vi "TestReadWrites.vi"() -> ()   [LabVIEW 2017]
uses:
  Global 1.vi
panel:
  in  "Indicator 2":dbl
  out "Array":dbl[][](array[numeric])
  out "Indicator":dbl
  out "Time per write":dbl[](array[numeric])
  in  "Iterations":i32=5000
  # "Control/Indicator"
  # "Local Variable"
  # "Property Node"
  # "Global Variable"
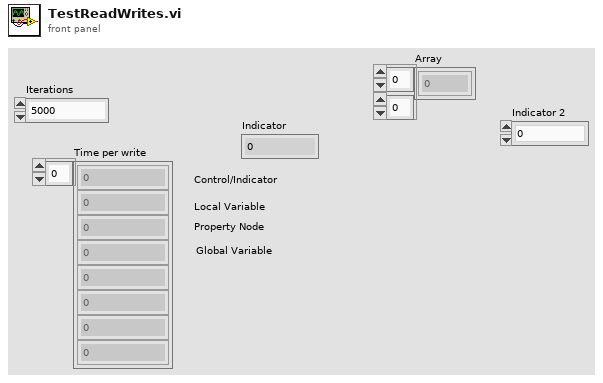
[diagram p1: front panel]
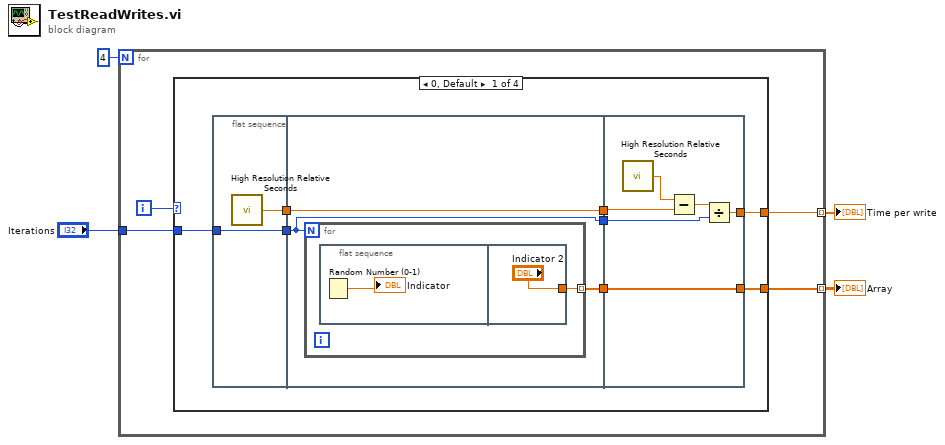
[diagram p0: block diagram]
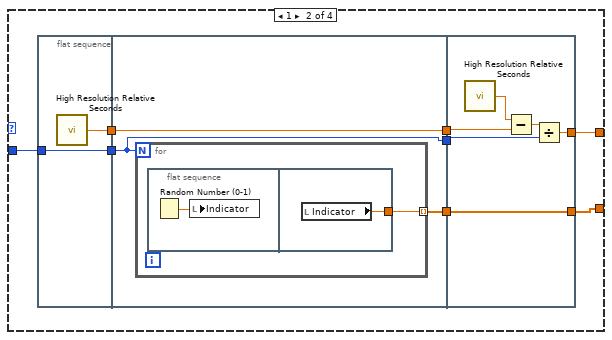
[diagram p2: hidden frame]
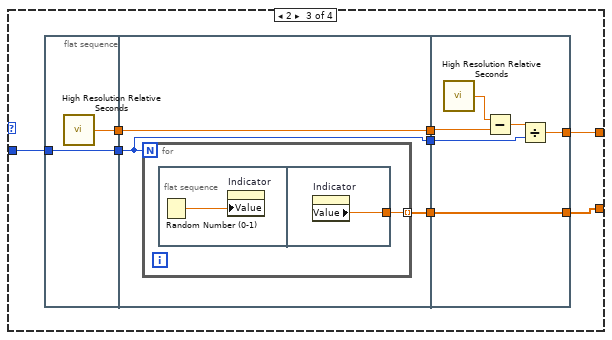
[diagram p3: hidden frame]
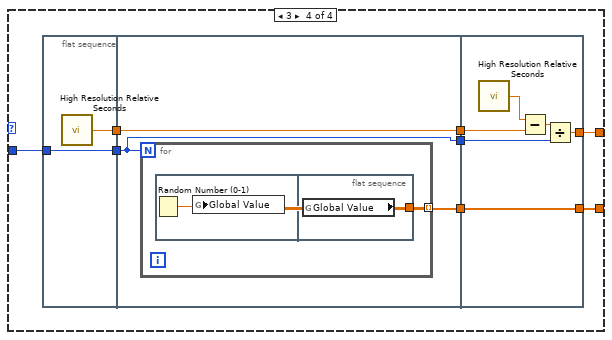
[diagram p4: hidden frame]
diagram:
  n1 = for {
    N: 4 -> [_]
    tunnel: "Iterations" -> [w7]
    tunnel: [w6] -> w3 mode=indexing
    tunnel: [w5] -> w1 mode=indexing
    i -> [w8]
    n2 = case shown="0, Default" w8 {
      tunnel: w7 -> [w14 w36 w58 w80]
      tunnel: [w11 w33 w55 w77] -> w6
      tunnel: [w10 w31 w54 w75] -> w5
      frame 0, Default {
        n3 = flat-sequence {
          tunnel: [w18] -> w15
          tunnel: w14 -> [w17]
          tunnel: [w17] -> w13
          tunnel: [w21] -> w16
          tunnel: w15 -> [w21]
          tunnel: w13 -> [w20]
          tunnel: [w20] -> w12
          tunnel: [w19] -> w9
          tunnel: w16 -> [w29]
          tunnel: w12 -> [w27]
          tunnel: [w26] -> w11
          tunnel: [w25] -> w10
          tunnel: w9 -> [w25]
          frame #0 {
            n4 = call <vilib>:"High Resolution Relative Seconds.vi"() -> ("relative seconds"=w18:dbl)
          }
          frame #1 {
            n5 = for {
              N: w20 -> [_]
              tunnel: [w22] -> w19 mode=indexing
              n6 = flat-sequence {
                tunnel: ["Indicator 2"] -> w22
                frame #0 {
                  n7 = Random Number (0-1)() -> (number: 0 to 1=→"Indicator":dbl)
                }
                frame #1 {
                }
              }
            }
          }
          frame #2 {
            n8 = call <vilib>:"High Resolution Relative Seconds.vi"() -> ("relative seconds"=w30:dbl)
            n9 = Subtract(x=w30, y=w29) -> (x-y=w28:dbl)
            n10 = Divide(x=w28, y=w27) -> (x/y=w26:dbl)
          }
        }
      }
      frame 1 {
        n11 = flat-sequence {
          tunnel: [w40] -> w37
          tunnel: w36 -> [w39]
          tunnel: [w39] -> w35
          tunnel: [w43] -> w38
          tunnel: w37 -> [w43]
          tunnel: w35 -> [w42]
          tunnel: [w42] -> w34
          tunnel: [w41] -> w32
          tunnel: w38 -> [w51]
          tunnel: w34 -> [w49]
          tunnel: [w48] -> w33
          tunnel: [w47] -> w31
          tunnel: w32 -> [w47]
          frame #0 {
            n12 = call <vilib>:"High Resolution Relative Seconds.vi"() -> ("relative seconds"=w40:dbl)
          }
          frame #1 {
            n13 = for {
              N: w42 -> [_]
              tunnel: [w44] -> w41 mode=indexing
              n14 = flat-sequence {
                tunnel: [w46] -> w44
                frame #0 {
                  n15 = Random Number (0-1)() -> (number: 0 to 1=w45:dbl)
                  n16 = local write "Indicator"(w45) -> ()
                }
                frame #1 {
                  n17 = local read "Indicator"() -> (w46:dbl)
                }
              }
            }
          }
          frame #2 {
            n18 = call <vilib>:"High Resolution Relative Seconds.vi"() -> ("relative seconds"=w52:dbl)
            n19 = Subtract(x=w52, y=w51) -> (x-y=w50:dbl)
            n20 = Divide(x=w50, y=w49) -> (x/y=w48:dbl)
          }
        }
      }
      frame 2 {
        n21 = flat-sequence {
          tunnel: [w62] -> w59
          tunnel: w58 -> [w61]
          tunnel: [w61] -> w57
          tunnel: [w65] -> w60
          tunnel: w59 -> [w65]
          tunnel: w57 -> [w64]
          tunnel: [w64] -> w56
          tunnel: [w63] -> w53
          tunnel: w60 -> [w73]
          tunnel: w56 -> [w71]
          tunnel: [w70] -> w55
          tunnel: [w69] -> w54
          tunnel: w53 -> [w69]
          frame #0 {
            n22 = call <vilib>:"High Resolution Relative Seconds.vi"() -> ("relative seconds"=w62:dbl)
          }
          frame #1 {
            n23 = for {
              N: w64 -> [_]
              tunnel: [w66] -> w63 mode=indexing
              n24 = flat-sequence {
                tunnel: [w68] -> w66
                frame #0 {
                  n25 = Random Number (0-1)() -> (number: 0 to 1=w67:dbl)
                  n26 = property on="Indicator" class="DigNum (strict)"("Value"=w67) -> ()  [unwired: 2 in, 2 out]
                }
                frame #1 {
                  n27 = property on="Indicator" class="DigNum (strict)"() -> ("Value"=w68:dbl)  [unwired: 2 in, 2 out]
                }
              }
            }
          }
          frame #2 {
            n28 = call <vilib>:"High Resolution Relative Seconds.vi"() -> ("relative seconds"=w74:dbl)
            n29 = Subtract(x=w74, y=w73) -> (x-y=w72:dbl)
            n30 = Divide(x=w72, y=w71) -> (x/y=w70:dbl)
          }
        }
      }
      frame 3 {
        n31 = flat-sequence {
          tunnel: [w84] -> w81
          tunnel: w80 -> [w83]
          tunnel: [w83] -> w79
          tunnel: [w87] -> w82
          tunnel: w81 -> [w87]
          tunnel: w79 -> [w86]
          tunnel: [w86] -> w78
          tunnel: [w85] -> w76
          tunnel: w82 -> [w95]
          tunnel: w78 -> [w93]
          tunnel: [w92] -> w77
          tunnel: w76 -> [w91]
          tunnel: [w91] -> w75
          frame #0 {
            n32 = call <vilib>:"High Resolution Relative Seconds.vi"() -> ("relative seconds"=w84:dbl)
          }
          frame #1 {
            n33 = for {
              N: w86 -> [_]
              tunnel: [w88] -> w85 mode=indexing
              n34 = flat-sequence {
                tunnel: [w90] -> w88
                frame #0 {
                  n35 = Random Number (0-1)() -> (number: 0 to 1=w89:dbl)
                  n36 = global write "Global 1.vi" "Global Value"(w89) -> ()
                }
                frame #1 {
                  n37 = global read "Global 1.vi" "Global Value"() -> (w90:dbl)
                }
              }
            }
          }
          frame #2 {
            n38 = call <vilib>:"High Resolution Relative Seconds.vi"() -> ("relative seconds"=w96:dbl)
            n39 = Subtract(x=w96, y=w95) -> (x-y=w94:dbl)
            n40 = Divide(x=w94, y=w93) -> (x/y=w92:dbl)
          }
        }
      }
    }
  }
  "Time per write" <- w3
  "Array" <- w1
